vi "FRCts20_Backend_API_TeamRoot.vi"(8 "error in (no error)":errorcluster, 10 "Command":T1="GetTeamRoot", 11 "Team In":T2) -> (0 "error out":errorcluster, 2 "Status":string, 3 "Team Out":T2)   [LabVIEW 2013, in "FRCts20_Backend_API.lvlib"]
doc: "This API call returns all team information or creates a new team"
uses:
  FRCts20_Backend_API.lvlib
  FRCts20_Backend_API_TeamRoot.ctl
  FRCts20_Backend_API_SW.ctl
  FRCts20_Backend_API_Command_TeamRoot.ctl
  FRCts20_Backend_FGVOperation.ctl
  FRCts20_Backend_Engine.lvlib
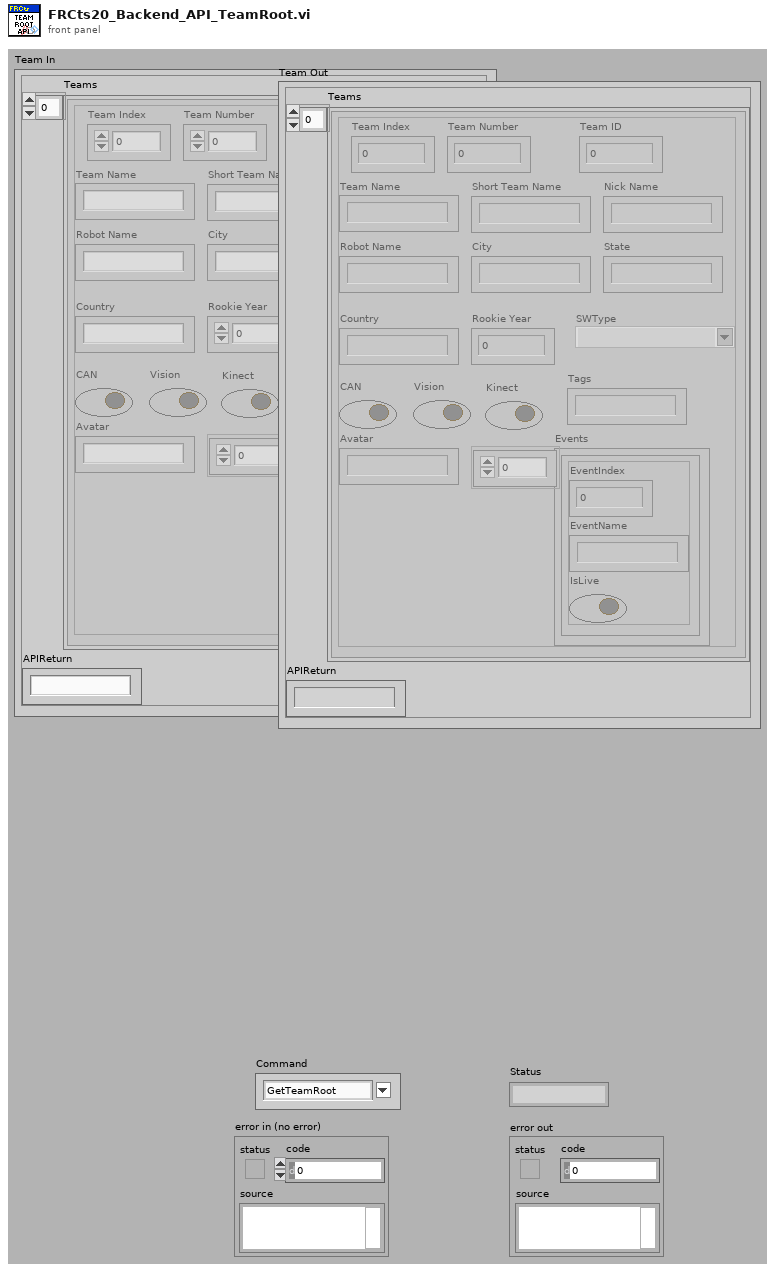
[diagram p1: front panel]
types:
  T1 = typedef "FRCts20_Backend_API.lvlib/FRCts20_Backend_API_Command_TeamRoot.ctl" = string
  T2 = typedef "FRCts20_Backend_API.lvlib/FRCts20_Backend_API_TeamRoot.ctl" = cluster{"Teams":cluster{"Team Index":u32, "Team Number":u32, "Team ID":u32, "Team Name":string, "Short Team Name":string, "Nick Name":string, "Robot Name":string, "City":string, "State":string, "Country":string, "Rookie Year":u32, "SWType":T3, "CAN":bool, "Vision":bool, "Kinect":bool, "Tags":string, "Avatar":string, "Events":cluster{"EventIndex":u32, "EventName":string, "IsLive":bool}[]}[], "APIReturn":string}
  T3 = typedef "FRCts20_Backend_API.lvlib/FRCts20_Backend_API_SW.ctl" = string
  T4 = typedef "FRCts20_Backend_Engine.lvlib/FRCts20_Backend_FGVOperation.ctl" = enum16{"Initialize", "EnqueueMessage", "EnqueueDataReturn", "FlushMessage", "FlushDataReturn"}
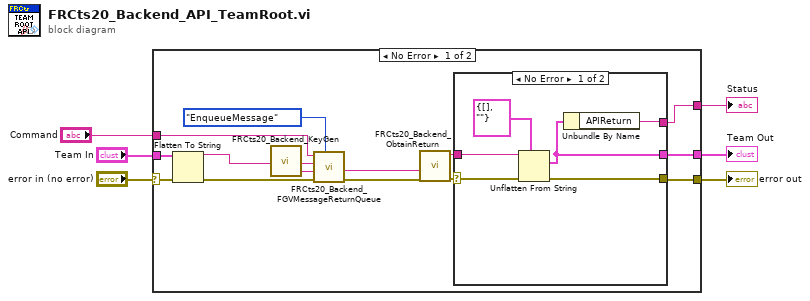
[diagram p0: block diagram]
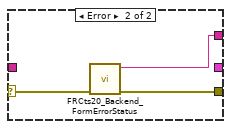
[diagram p2: hidden frame]
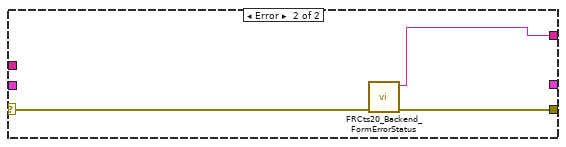
[diagram p3: hidden frame]
diagram:
  n1 = case shown="No Error" "error in (no error)" {
    selector: "error in (no error)" -> [w19 w30]
    tunnel: [w7 w31] -> w5
    tunnel: [w9 w32] -> w4
    tunnel: "Command" -> [w13 _]
    tunnel: "Team In" -> [w12 _]
    tunnel: [w8 _] -> w2
    frame No Error {
      n2 = Flatten To String(anything=w12, error in (no error)=w19) -> (data string=w20:string, error out=w18:errorcluster)  [unwired: 2 in, 1 out]
      n3 = call "FRCts20_Backend_KeyGen.vi"() -> ("Keygen"=w17:string)  [unwired: 27 in]
      n4 = call "FRCts20_Backend_FGVMessageReturnQueue.vi"("Operation"=FRCts20_Backend_FGVOperation."EnqueueMessage", "error in (no error)"=w18, "Key"=w17, "Message Value"=w20, "Message Name"=w13) -> ("error out"=w15:errorcluster, "Key (Duplicate)"=w14:string)  [unwired: 5 in]
      n5 = call "FRCts20_Backend_ObtainReturn.vi"("error in (no error)"=w15, "Key"=w14) -> ("error out"=w11:errorcluster, "Message Value"=w10:string)  [unwired: 8 in]
      n6 = case shown="No Error" w11 {
        selector: w11 -> [w25 w29]
        tunnel: [w26 w28] -> w7
        tunnel: [w24 _] -> w8
        tunnel: [w23 w27] -> w9
        tunnel: w10 -> [w22 _]
        frame No Error {
          n7 = Unflatten From String(type=T2 {"Teams"=[], "APIReturn"=""} ("Team Root"), binary string=w22, error in (no error)=w25) -> (value=w24:T2, error out=w26:errorcluster)  [unwired: 2 in, 1 out]
          n8 = Unbundle By Name(w24) -> ("APIReturn"=w23:string)
        }
        frame Error {
          n9 = call "FRCts20_Backend_FormErrorStatus.vi"("error in (no error)"=w29) -> ("error out"=w28:errorcluster, "String"=w27:string)  [unwired: 9 in]
        }
      }
    }
    frame Error {
      n10 = call "FRCts20_Backend_FormErrorStatus.vi"("error in (no error)"=w30) -> ("error out"=w31:errorcluster, "String"=w32:string)  [unwired: 9 in]
    }
  }
  "error out" <- w5
  "Status" <- w4
  "Team Out" <- w2
